vi "GetPmuImpairFrontPanel.vi"(8 "ErrorArray In":errorcluster[](array[cluster]), 11 "Bus.lvclass In":refnum<class "Bus.lvclass">) -> (0 "ErrorArray Out":errorcluster[](array[cluster]), 3 "Bus.lvclass Out":refnum<class "Bus.lvclass">)   [LabVIEW 2017, in "Bus_class.lvlib" / "Bus.lvclass"]
uses:
  Bus.lvclass
  Framework.lvlib
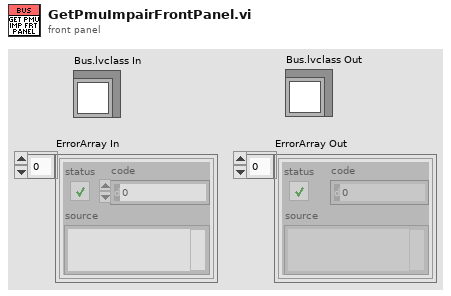
[diagram p1: front panel]
types:
  T1 = typedef "Framework.lvlib/clFrontPanelControlRefs.ctl" = cluster{"TestFilePathRef":refnum<vi>, "BusNumberRef":refnum<vi>, "NumberOfBusesRef":refnum<vi>, "EvtTypeRef":refnum<vi>, "EvtParamsRef":refnum<vi>, "EvtConfigRef":refnum<vi>, "StartTimeRef":refnum<vi>, "EndTimeRef":refnum<vi>, "PmuImpairTypeRef":refnum<vi>, "PmuImpairParamsRef":refnum<vi>, "NetImpairParamsRef":refnum<vi>, "FlagImpairTypeRef":refnum<vi>, "FlagImpairParamsRef":refnum<vi>, "NetImpairTypeRef":refnum<vi>, "OutputFileType":refnum<vi>, "PmuImpairConfigRef":refnum<vi>, "AppTypeRef":refnum<vi>, "ScriptPathRef":refnum<vi>, "ShowPanels?":refnum<vi>}
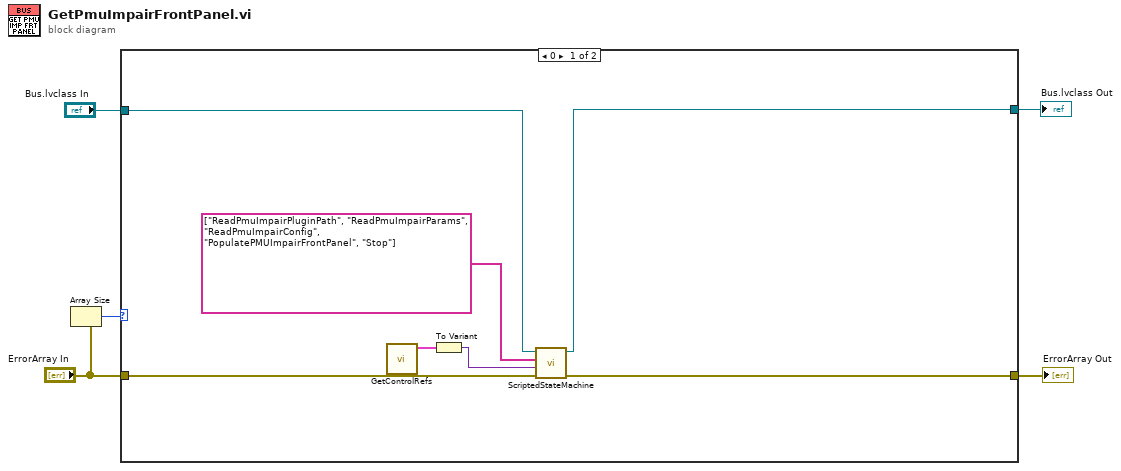
[diagram p0: block diagram]
diagram:
  n1 = Array Size(array="ErrorArray In") -> (size(s)=w4:i32)
  n2 = case shown="0" w4 {
    tunnel: [w12 w14] -> w5
    tunnel: "ErrorArray In" -> [w10 w14]
    tunnel: "Bus.lvclass In" -> [w11 w13]
    tunnel: [w9 w13] -> w1
    frame 0 {
      n3 = call "GetControlRefs.vi"() -> ("clControlRefs Out"=w6:T1)  [unwired: 11 in]
      n4 = To Variant(anything=w6) -> (Variant=w7:variant)
      n5 = call "ScriptedStateMachine.vi"("ErrorArray In"=w10, "Data in"=w7, "Script"=string[] ["ReadPmuImpairPluginPath", "ReadPmuImpairParams", "ReadPmuImpairConfig", "PopulatePMUImpairFrontPanel", "Stop"], "Bus"=w11) -> ("ErrorArray Out"=w12:errorcluster[], "Bus"=w9:refnum<class "Bus.lvclass">)  [unwired: 5 in, 1 out]
    }
    frame 1, Default {
    }
  }
  "ErrorArray Out" <- w5
  "Bus.lvclass Out" <- w1
